vi "stop button.vi"() -> ()   [LabVIEW 2017]
panel:
  in  "ID":dbl
  in  "stop":bool
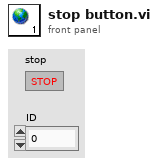
[diagram p1: front panel]
diagram:
